vi "SR830 sweep update tw temporary 4.vi"() -> ()   [LabVIEW 2015]
uses:
  magnetometers/smi/labview/CPM20Software/SmartMotor.llb/SM Config.ctl
  magnetometers/smi/labview/CPM20Software/SmartMotor.llb/SM MotorConfig.ctl
  <vilib>/Analysis/1siggen.llb/Ramp Pattern by Samples.vi
  <vilib>/Utility/file.llb/Write To Spreadsheet File (DBL).vi
  Global vab.vi
  <vilib>/Analysis/NI_AALBase.lvlib
panel:
  in  "Laser lock":bool
  out "read buffer":string
  in  "USB relay com port":refnum<visa-resource-name>="COM5"
  in  "Back position (mm)":dbl=120.0
  in  "Back velocity (mm/sec)":dbl=1.0
  out "SM motor moving":bool
  out "Lock data":dbl[][](array[numeric])=[[0.0, -9.2798e-08], [0.0, -9.27907e-08], [0.0, -9.27762e-08], [0.00508, -9.27762e-08], [0.03048, -9.27762e-08], [0.10668000000000001, -9.27762e-08], [0.17272, -9.27762e-08], [0.23368, -9.27762e-08], [0.28956000000000004, -9.27253e-08], [0.34036000000000005, -9.27253e-08], [0.39116, -9.27325e-08], [0.43688, -9.27398e-08], [0.48768, -9.27398e-08], [0.5334, -9.27253e-08], [0.5842, -9.2718e-08], [0.635, -9.27253e-08], [0.6807200000000001, -9.27253e-08], [0.73152, -9.27107e-08], [0.78232, -9.27034e-08], [0.8331200000000001, -9.2718e-08], [0.8839199999999999, -9.2718e-08], [0.93472, -9.27398e-08], [0.9855200000000001, -9.27253e-08], [1.0312400000000002, -9.2718e-08], [1.08204, -9.27253e-08], [1.12776, -9.27253e-08], [1.17856, -9.2718e-08], [1.22936, -9.2718e-08], [1.27508, -9.2718e-08], [1.3258800000000002, -9.27253e-08], [1.3766800000000001, -9.27471e-08], [1.4224, -9.27544e-08], [1.4731999999999998, -9.27471e-08], [1.524, -9.27398e-08], [1.56972, -9.27398e-08], [1.6256000000000002, -9.27471e-08], [1.6713200000000001, -9.27398e-08], [1.72212, -9.27398e-08], [1.7729199999999998, -9.27398e-08], [1.81864, -9.27398e-08], [1.86944, -9.27325e-08], [1.91516, -9.27398e-08], [1.9659600000000002, -9.27471e-08], [2.01168, -9.27325e-08], [2.0624800000000003, -9.27325e-08], [2.11836, -9.27544e-08], [2.16408, -9.27398e-08], [2.21488, -9.27398e-08], [2.2606, -9.27253e-08], [2.3114, -9.27253e-08], [2.35712, -9.2718e-08], [2.40792, -9.27253e-08], [2.45364, -9.27253e-08], [2.50444, -9.2718e-08], [2.55524, -9.27398e-08], [2.60604, -9.27325e-08], [2.6568400000000003, -9.26962e-08], [2.70764, -9.26743e-08], [2.7584400000000002, -9.26889e-08], [2.8092400000000004, -9.2718e-08], [2.8600399999999997, -9.2718e-08], [2.90576, -9.2718e-08], [2.9514799999999997, -9.2718e-08], [3.00228, -9.2718e-08], [3.048, -9.26889e-08], [3.0987999999999998, -9.26816e-08], [3.1496, -9.27034e-08], [3.2004, -9.2718e-08], [3.24612, -9.2718e-08], [3.29184, -9.2718e-08], [3.3426400000000003, -9.2718e-08], [3.3934400000000005, -9.27107e-08], [3.44424, -9.26889e-08], [3.49504, -9.26598e-08], [3.5509199999999996, -9.26743e-08], [3.59664, -9.27107e-08], [3.64744, -9.2718e-08], [3.6982399999999997, -9.27107e-08], [3.73888, -9.2718e-08], [3.79476, -9.27107e-08], [3.84048, -9.27325e-08], [3.89128, -9.27253e-08], [3.9370000000000003, -9.27253e-08], [3.9878, -9.2718e-08], [4.03352, -9.27107e-08], [4.08432, -9.2718e-08], [4.13512, -9.2718e-08], [4.18084, -9.27107e-08], [4.23164, -9.27107e-08], [4.28244, -9.2718e-08], [4.33832, -9.27398e-08], [4.37896, -9.27398e-08], [4.42976, -9.27253e-08], [4.48056, -9.2718e-08], [4.52628, -9.2718e-08], [4.5770800000000005, -9.2718e-08], [4.6228, -9.27034e-08], [4.6736, -9.26962e-08], [4.7244, -9.26889e-08], [4.7701199999999995, -9.26962e-08], [4.82092, -9.27034e-08], [4.87172, -9.2718e-08], [4.91744, -9.2718e-08], [4.97332, -9.27107e-08], [5.0038, -9.27107e-08], [0.0, -9.27253e-08], [4.99872, -9.27253e-08], [4.99872, -9.27253e-08], [4.99872, -9.2718e-08], [4.94284, -9.27034e-08], [4.86156, -9.26889e-08], [4.8006, -9.26743e-08], [4.74472, -9.26743e-08], [4.69392, -9.26962e-08], [4.643120000000001, -9.27034e-08], [4.59232, -9.26962e-08], [4.5466, -9.27034e-08], [4.4958, -9.27107e-08], [4.45008, -9.27034e-08], [4.40436, -9.26962e-08], [4.35356, -9.26816e-08], [4.30784, -9.27034e-08], [4.2621199999999995, -9.26962e-08], [4.2164, -9.26889e-08], [4.17068, -9.27034e-08], [4.11988, -9.27034e-08], [4.07924, -9.27034e-08], [4.02336, -9.26962e-08], [3.97764, -9.26598e-08], [3.9268400000000003, -9.26816e-08], [3.88112, -9.27034e-08], [3.8354, -9.26889e-08], [3.78968, -9.26962e-08], [3.73888, -9.26889e-08], [3.6931599999999998, -9.26889e-08], [3.64744, -9.27107e-08], [3.59664, -9.2718e-08], [3.5559999999999996, -9.27471e-08], [3.5052, -9.27471e-08], [3.45948, -9.27398e-08], [3.4137600000000003, -9.2718e-08], [3.36804, -9.2718e-08], [3.3223200000000004, -9.27253e-08], [3.27152, -9.27325e-08], [3.2258, -9.27253e-08], [3.1800800000000002, -9.27253e-08], [3.13436, -9.2718e-08], [3.0734, -9.27107e-08], [3.03276, -9.26816e-08], [2.98704, -9.26962e-08], [2.9362399999999997, -9.27034e-08], [2.89052, -9.2718e-08], [2.84988, -9.2718e-08], [2.7940000000000005, -9.26671e-08], [2.7533600000000003, -9.26743e-08], [2.70764, -9.26962e-08], [2.6568400000000003, -9.27107e-08], [2.61112, -9.27034e-08], [2.5654, -9.27034e-08], [2.5146, -9.26816e-08], [2.46888, -9.26743e-08], [2.4231599999999998, -9.26816e-08], [2.37744, -9.27034e-08], [2.3266400000000003, -9.27107e-08], [2.28092, -9.27034e-08], [2.2352, -9.2718e-08], [2.1844, -9.2718e-08], [2.13868, -9.27034e-08], [2.0929599999999997, -9.27034e-08], [2.04216, -9.27034e-08], [1.99136, -9.27034e-08], [1.95072, -9.26962e-08], [1.905, -9.26816e-08], [1.85928, -9.26816e-08], [1.8084799999999999, -9.26889e-08], [1.7627599999999999, -9.26889e-08], [1.7170400000000001, -9.26962e-08], [1.6662400000000002, -9.27034e-08], [1.62052, -9.27107e-08], [1.5748, -9.2718e-08], [1.52908, -9.2718e-08], [1.4731999999999998, -9.2718e-08], [1.4325599999999998, -9.27107e-08], [1.38684, -9.2718e-08], [1.3360400000000001, -9.27107e-08], [1.28524, -9.26962e-08], [1.2446, -9.26962e-08], [1.19888, -9.26962e-08], [1.14808, -9.26962e-08], [1.10236, -9.27107e-08], [1.05664, -9.27107e-08], [1.01092, -9.27253e-08], [0.96012, -9.27253e-08], [0.9144, -9.2718e-08], [0.8636, -9.2718e-08], [0.81788, -9.27253e-08], [0.77216, -9.2718e-08], [0.72644, -9.2718e-08], [0.67564, -9.27034e-08], [0.62992, -9.27107e-08], [0.5791200000000001, -9.27253e-08], [0.52832, -9.2718e-08], [0.48768, -9.2718e-08], [0.44195999999999996, -9.27034e-08], [0.39624, -9.26962e-08], [0.35052000000000005, -9.27034e-08], [0.30988, -9.26889e-08], [0.26416, -9.26743e-08], [0.21844, -9.26889e-08], [0.17272, -9.26889e-08], [0.127, -9.26889e-08], [0.09652, -9.26889e-08], [0.04064, -9.26962e-08], [-0.00508, -9.26962e-08], [0.0, -9.27544e-08]]
  out "Last lock file":path=path "C:/Shoujun/07272005/lock.008"
  in  "Save lock":bool
  out "Last sweep file":path=path "C:/Shoujun/06122015/scan002"
  in  "Save sweep":bool
  out "Ccurrent times":dbl
  in  "Moving times":dbl=1.0
  in  "Waiting time (s)":dbl=3.0
  in  "Stop motor":bool
  out "Motor position (mm)":dbl
  in  "SM setting":T1={"Acceleration (mm/sec^2)"=1000.0, "Velocity (mm/sec)"=2.0, "Position (mm)"=0.0} {"Position (mm)" format="%.3f"; "Velocity (mm/sec)" format="%.3f"; "Acceleration (mm/sec^2)" format="%.3f"}
  in  "SM Config":T2={"VISA Serial ref"="COM3", "Motor Config"={"DriveRatio (mm/rev)"=10.16, "PosLimit + (mm)"=200.0, "PosLimit - (mm)"=0.0, "EncoderRatio (count/rev)"=2000.0, "MotorType"=enum."SM17"}} {"Motor Config"."EncoderRatio (count/rev)" format="%.2f"; "Motor Config"."PosLimit - (mm)" format="%.3f"; "Motor Config"."PosLimit + (mm)" format="%.3f"; "Motor Config"."DriveRatio (mm/rev)" format="%.2f"}
  in  "Motor moving mode":u16(ring) items=["One-way", "Two-way"]
  out "Step time (ms)":u32
  out "Center Freq. (Hz)":dbl=1279.6242713207916 format="%#_8f"
  in  "DS345 parameters":T4={"Osc. Amp. (V)"=0.06, "Osc. Freq. (Hz)"=1140.0} {"Osc. Freq. (Hz)" min=0.001 max=250000.0 step=0.001 format="%.3f"; "Osc. Amp. (V)" min=0.0 max=0.1 step=0.001 format="%.3f"}
  out "Lock Chart":dbl(graph)
  in  "Lock":bool
  in  "Update":bool
  in  "Auto-phase":bool
  in  "Update Aux Outs":bool
  in  "Lock-in  \naux outs (V)":dbl[](array[numeric])=[3.0, 0.0, -3.0, 4.0]
  in  "stop":bool
  in  "Lock in parameters":T5={"Phase (deg)"=190.0, "TC"=7, "TC Multiplier"=5.0} {"TC Multiplier" min=0.0 max=10.0 step=1.0 format="%.2f"; "TC" items=["10 µs", "30 µs", "100 µs", "300 µs", "1 ms", "3 ms", "10 ms", "30 ms", "100 ms", "300 ms", "1 s", "3 s", "10 s", "30 s", "100 s", "300 s", "1 ks", "3 ks", "10 ks", "30 ks"]; "Phase (deg)" format="%.3f"}
  out "Sweep Fit Chart":dbl[][](graph)
  out "Best Fit Coefficients":dbl[][](array[numeric])=[[116.36223046164876, 1127.5591284236862, 2.415453805851806, 2.8898288492774762e-08, 1.3970935970960048e-10, -9.348733573586501e-08], [116.33952287251303, 1126.8840669250824, 92.71773761789645, 2.8818113222476787e-08, 1.0278120537649892e-10, 1.3998320692235225e-07]] format="%#_6p"
  out "Sweep fit data":dbl[][](array[numeric])=[[-9.278428993694947e-08, 1.2151206747589936e-07], [-9.257777429927783e-08, 1.2146574495873341e-07], [-9.237209921929236e-08, 1.2141607252254236e-07], [-9.216734571334164e-08, 1.2136297955084925e-07], [-9.196359932316975e-08, 1.2130639502797934e-07], [-9.176095032811043e-08, 1.2124624766638154e-07], [-9.155949396397681e-08, 1.2118246604883246e-07], [-9.13593306484252e-08, 1.211149787867336e-07], [-9.116056621249537e-08, 1.2104371469578182e-07], [-9.096331213794347e-08, 1.2096860299036584e-07], [-9.076768579988502e-08, 1.208895734981137e-07], [-9.057381071415596e-08, 1.2080655689608598e-07], [-9.038181678867532e-08, 1.2071948497018084e-07], [-9.019184057795565e-08, 1.2062829089938097e-07], [-9.000402553975253e-08, 1.2053290956653703e-07], [-8.98185222926743e-08, 1.20433277897436e-07], [-8.963548887338411e-08, 1.203293352299526e-07], [-8.945509099181811e-08, 1.2022102371511948e-07], [-8.92775022826158e-08, 1.2010828875197835e-07], [-8.910290455070839e-08, 1.1999107945808357e-07], [-8.893148800873977e-08, 1.1986934917752383e-07], [-8.876345150369997e-08, 1.1974305602829554e-07], [-8.859900272983336e-08, 1.1961216349080777e-07], [-8.843835842454211e-08, 1.1947664103921127e-07], [-8.828174454364171e-08, 1.193364648171232e-07], [-8.812939641193772e-08, 1.1919161835915823e-07], [-8.798155884468516e-08, 1.1904209335946764e-07], [-8.783848623506419e-08, 1.1888789048822932e-07], [-8.770044260236139e-08, 1.1872902025671231e-07], [-8.756770159508958e-08, 1.1856550393115542e-07], [-8.744054644281251e-08, 1.1839737449524304e-07], [-8.731926984997504e-08, 1.1822467766042538e-07], [-8.720417382457544e-08, 1.1804747292270706e-07], [-8.709556943406905e-08, 1.1786583466381296e-07], [-8.699377648046863e-08, 1.1767985329382321e-07], [-8.689912308622005e-08, 1.1748963643144947e-07], [-8.681194518209715e-08, 1.1729531011709283e-07], [-8.673258588809238e-08, 1.1709702005268066e-07], [-8.66613947780996e-08, 1.1689493286102198e-07], [-8.659872701911271e-08, 1.166892373560515e-07], [-8.654494237572095e-08, 1.1648014581385351e-07], [-8.650040407089468e-08, 1.162678952327797e-07], [-8.646547749444962e-08, 1.1605274856930732e-07], [-8.644052875118079e-08, 1.1583499593454794e-07], [-8.64259230414993e-08, 1.1561495573452977e-07], [-8.642202286851262e-08, 1.1539297573557164e-07], [-8.642918606689061e-08, 1.1516943403427588e-07], [-8.644776365058209e-08, 1.1494473990993435e-07], [-8.64780974785094e-08, 1.1471933453551767e-07], [-8.652051773979436e-08, 1.1449369152195575e-07], [-8.657534026286338e-08, 1.1426831726918777e-07], [-8.664286365595156e-08, 1.140437510965259e-07], [-8.672336629006395e-08, 1.138205651243217e-07], [-8.681710313934008e-08, 1.1359936387882222e-07], [-8.692430249797145e-08, 1.1338078359254025e-07], [-8.704516259729139e-08, 1.131654911735182e-07], [-8.717984815132624e-08, 1.129541828186175e-07], [-8.73284868638809e-08, 1.1274758224848306e-07], [-8.749116593502439e-08, 1.125464385451754e-07], [-8.766792860952055e-08, 1.123515235776711e-07], [-8.785877081417203e-08, 1.1216362900552807e-07], [-8.80636379350548e-08, 1.1198356285698996e-07], [-8.828242178904716e-08, 1.1181214568462754e-07], [-8.851495784672179e-08, 1.1165020630921665e-07], [-8.87610227653934e-08, 1.1149857717082398e-07], [-8.902033229172319e-08, 1.1135808931486821e-07], [-8.92925395926122e-08, 1.112295670500614e-07], [-8.957723407103051e-08, 1.1111382232439058e-07], [-8.987394071981971e-08, 1.1101164887441855e-07], [-9.018212006130215e-08, 1.1092381621188385e-07], [-9.050116871371693e-08, 1.108510635195627e-07], [-9.08304206171131e-08, 1.1079409353531224e-07], [-9.116914894146363e-08, 1.1075356650884374e-07], [-9.151656868858414e-08, 1.1073009431979129e-07], [-9.187183998717035e-08, 1.107242348477972e-07], [-9.22340720671979e-08, 1.1073648668542749e-07], [-9.260232788639432e-08, 1.107672842826178e-07], [-9.297562936787966e-08, 1.1081699360696361e-07], [-9.335296319478886e-08, 1.1088590839752084e-07], [-9.373328709516066e-08, 1.109742470809708e-07], [-9.411553653902002e-08, 1.1108215040820914e-07], [-9.449863175978703e-08, 1.1120967985690896e-07], [-9.488148500426463e-08, 1.1135681683171895e-07], [-9.526300790977496e-08, 1.1152346267888724e-07], [-9.564211890374562e-08, 1.117094395166938e-07], [-9.601775052031209e-08, 1.1191449186759197e-07], [-9.638885653034085e-08, 1.1213828906287883e-07], [-9.675441878561362e-08, 1.1238042837648129e-07], [-9.711345368460556e-08, 1.1264043883148628e-07], [-9.746501817608558e-08, 1.1291778561171267e-07], [-9.780821522736294e-08, 1.1321187500122058e-07], [-9.814219869602744e-08, 1.1352205976739033e-07], [-9.84661775570772e-08, 1.1384764489820865e-07], [-9.877941945096975e-08, 1.1418789360171566e-07], [-9.908125353194587e-08, 1.1454203347514908e-07], [-9.937107260954993e-08, 1.1490926275305287e-07], [-9.964833458923416e-08, 1.1528875654731036e-07], [-9.991256322995798e-08, 1.1567967299747591e-07], [-1.0016334824750823e-07, 1.1608115925663376e-07], [-1.0040034480166377e-07, 1.164923572460048e-07], [-1.0062327241316715e-07, 1.1691240912033472e-07], [-1.0083191336266948e-07, 1.173404623954193e-07], [-1.0102611062836781e-07, 1.177756746986579e-07], [-1.0120576542199472e-07, 1.1821721811300182e-07], [-1.0137083438423545e-07, 1.1866428309384035e-07], [-1.0152132650066499e-07, 1.191160819470443e-07], [-1.0165729979806487e-07, 1.1957185186439482e-07], [-1.0177885787867792e-07, 1.2003085751985298e-07], [-1.0188614634676502e-07, 1.2049239323648097e-07], [-1.0197934917793213e-07, 1.2095578473926653e-07], [-1.0205868507727816e-07, 1.2142039051361878e-07], [-1.0212440386764666e-07, 1.2188560279290256e-07], [-1.0217678294430411e-07, 1.223508482011107e-07], [-1.0221612382735416e-07, 1.228155880786833e-07], [-1.0224274883825146e-07, 1.232793185206537e-07], [-1.0225699792200032e-07, 1.2374157015680308e-07], [-1.0225922563209356e-07, 1.2420190770342955e-07], [-1.0224979829102574e-07, 1.2465992931576863e-07], [-1.0222909133534692e-07, 1.251152657691261e-07], [-1.0219748685073481e-07, 1.2556757949547977e-07], [-1.0215537129946893e-07, 1.2601656350075602e-07], [-1.0210313343999116e-07, 1.2646194018625233e-07], [-1.0204116243592457e-07, 1.269034600958256e-07], [-1.0196984614998213e-07, 1.2734090060854922e-07], [-1.0188956961660426e-07, 1.2777406459460899e-07], [-1.0180071368589654e-07, 1.2820277905029003e-07], [-1.0170365383046482e-07, 1.2862689372604844e-07], [-1.0159875910603566e-07, 1.2904627975987226e-07], [-1.014863912562747e-07, 1.2946082832644712e-07], [-1.0136690395194417e-07, 1.2987044931105887e-07], [-1.012406421544441e-07, 1.3027507001570074e-07], [-1.0110794159383338e-07, 1.3067463390350941e-07], [-1.0096912835159999e-07, 1.3106909938643534e-07], [-1.0082451853872258e-07, 1.3145843865995573e-07], [-1.0067441805991713e-07, 1.3184263658765976e-07], [-1.0051912245537246e-07, 1.3222168963767397e-07], [-1.0035891681173344e-07, 1.325956048721376e-07], [-1.0019407573457405e-07, 1.3296439899028532e-07], [-1.0002486337510369e-07, 1.3332809742513234e-07], [-9.985153350435836e-08, 1.3368673349328222e-07], [-9.967432962863503e-08, 1.3404034759698076e-07], [-9.949348514042729e-08, 1.343889864772119e-07], [-9.930922349960456e-08, 1.347327025163688e-07], [-9.912175844004607e-08, 1.350715530888238e-07], [-9.893129419738688e-08, 1.3540559995756362e-07], [-9.873802575395663e-08, 1.3573490871493906e-07], [-9.854213909739125e-08, 1.360595482655007e-07], [-9.834381148977033e-08, 1.3637959034884478e-07], [-9.814321174448147e-08, 1.3669510910037385e-07], [-9.794050050833378e-08, 1.3700618064788107e-07]] format="%#_6p"
  out "Sweep data":dbl[][](array[numeric])=[[1040.0, -9.17285e-08, 1.21029e-07], [1041.0738255033557, -9.19904e-08, 1.21277e-07], [1042.1476510067114, -9.20122e-08, 1.21306e-07], [1043.221476510067, -9.20268e-08, 1.2132e-07], [1044.2953020134228, -9.19831e-08, 1.21277e-07], [1045.3691275167785, -9.19758e-08, 1.21262e-07], [1046.4429530201342, -9.18303e-08, 1.21269e-07], [1047.5167785234898, -9.16557e-08, 1.21233e-07], [1048.5906040268455, -9.14592e-08, 1.21197e-07], [1049.6644295302012, -9.12628e-08, 1.21131e-07], [1050.7382550335572, -9.10227e-08, 1.21022e-07], [1051.8120805369128, -9.08117e-08, 1.20935e-07], [1052.8859060402685, -9.06152e-08, 1.20825e-07], [1053.9597315436242, -9.03897e-08, 1.20716e-07], [1055.03355704698, -9.0135e-08, 1.20578e-07], [1056.1073825503356, -8.9924e-08, 1.20462e-07], [1057.1812080536913, -8.97567e-08, 1.20389e-07], [1058.255033557047, -8.96111e-08, 1.20323e-07], [1059.3288590604027, -8.94511e-08, 1.20243e-07], [1060.4026845637584, -8.92619e-08, 1.20112e-07], [1061.476510067114, -8.90436e-08, 1.19931e-07], [1062.5503355704698, -8.88181e-08, 1.19763e-07], [1063.6241610738255, -8.86071e-08, 1.19603e-07], [1064.6979865771812, -8.84324e-08, 1.19443e-07], [1065.7718120805368, -8.82869e-08, 1.19327e-07], [1066.8456375838925, -8.81341e-08, 1.19144e-07], [1067.9194630872482, -8.78867e-08, 1.18941e-07], [1068.993288590604, -8.77194e-08, 1.1873e-07], [1070.0671140939598, -8.75593e-08, 1.18562e-07], [1071.1409395973155, -8.74502e-08, 1.18424e-07], [1072.2147651006712, -8.73192e-08, 1.18264e-07], [1073.288590604027, -8.72246e-08, 1.18097e-07], [1074.3624161073826, -8.71446e-08, 1.17995e-07], [1075.4362416107383, -8.70791e-08, 1.179e-07], [1076.510067114094, -8.69991e-08, 1.17769e-07], [1077.5838926174497, -8.69045e-08, 1.17602e-07], [1078.6577181208054, -8.68026e-08, 1.17369e-07], [1079.731543624161, -8.66571e-08, 1.17063e-07], [1080.8053691275168, -8.65844e-08, 1.16838e-07], [1081.8791946308725, -8.65043e-08, 1.16656e-07], [1082.9530201342282, -8.64825e-08, 1.16445e-07], [1084.0268456375838, -8.64388e-08, 1.16256e-07], [1085.1006711409395, -8.6417e-08, 1.16045e-07], [1086.1744966442952, -8.63806e-08, 1.15834e-07], [1087.248322147651, -8.63588e-08, 1.15594e-07], [1088.3221476510066, -8.63442e-08, 1.1539e-07], [1089.3959731543623, -8.63588e-08, 1.1515e-07], [1090.4697986577182, -8.64097e-08, 1.1499e-07], [1091.543624161074, -8.65043e-08, 1.14851e-07], [1092.6174496644296, -8.65407e-08, 1.14633e-07], [1093.6912751677853, -8.65844e-08, 1.14364e-07], [1094.765100671141, -8.66207e-08, 1.14109e-07], [1095.8389261744967, -8.66717e-08, 1.1384e-07], [1096.9127516778524, -8.67735e-08, 1.13571e-07], [1097.986577181208, -8.69118e-08, 1.13382e-07], [1099.0604026845638, -8.70646e-08, 1.13171e-07], [1100.1342281879195, -8.7181e-08, 1.12923e-07], [1101.2080536912752, -8.73265e-08, 1.12734e-07], [1102.2818791946308, -8.75084e-08, 1.1256e-07], [1103.3557046979865, -8.7683e-08, 1.12341e-07], [1104.4295302013422, -8.78285e-08, 1.12072e-07], [1105.503355704698, -8.80323e-08, 1.11883e-07], [1106.5771812080536, -8.82796e-08, 1.1173e-07], [1107.6510067114093, -8.85343e-08, 1.11592e-07], [1108.724832214765, -8.8738e-08, 1.1141e-07], [1109.7986577181207, -8.89927e-08, 1.11199e-07], [1110.8724832214766, -8.92546e-08, 1.11075e-07], [1111.9463087248323, -8.9582e-08, 1.1101e-07], [1113.020134228188, -8.99386e-08, 1.11002e-07], [1114.0939597315437, -9.02514e-08, 1.10981e-07], [1115.1677852348994, -9.05789e-08, 1.10901e-07], [1116.241610738255, -9.08917e-08, 1.10806e-07], [1117.3154362416108, -9.12191e-08, 1.10777e-07], [1118.3892617449665, -9.15975e-08, 1.10821e-07], [1119.4630872483222, -9.19904e-08, 1.1085e-07], [1120.5369127516778, -9.23615e-08, 1.10886e-07], [1121.6107382550335, -9.2718e-08, 1.10871e-07], [1122.6845637583892, -9.30454e-08, 1.10893e-07], [1123.758389261745, -9.3431e-08, 1.11002e-07], [1124.8322147651006, -9.3773e-08, 1.11046e-07], [1125.9060402684563, -9.41295e-08, 1.11082e-07], [1126.979865771812, -9.44933e-08, 1.11213e-07], [1128.0536912751677, -9.48717e-08, 1.11366e-07], [1129.1275167785234, -9.52136e-08, 1.11483e-07], [1130.2013422818793, -9.55774e-08, 1.11628e-07], [1131.275167785235, -9.59412e-08, 1.11883e-07], [1132.3489932885907, -9.63632e-08, 1.1213e-07], [1133.4228187919464, -9.67343e-08, 1.12399e-07], [1134.496644295302, -9.70836e-08, 1.12669e-07], [1135.5704697986578, -9.74401e-08, 1.12938e-07], [1136.6442953020135, -9.78184e-08, 1.13302e-07], [1137.7181208053692, -9.81458e-08, 1.13556e-07], [1138.7919463087248, -9.84296e-08, 1.13833e-07], [1139.8657718120805, -9.87279e-08, 1.14168e-07], [1140.9395973154362, -9.90044e-08, 1.14451e-07], [1142.013422818792, -9.92809e-08, 1.14844e-07], [1143.0872483221476, -9.96083e-08, 1.1523e-07], [1144.1610738255033, -9.98994e-08, 1.15695e-07], [1145.234899328859, -1.00161e-07, 1.16103e-07], [1146.3087248322147, -1.00423e-07, 1.16503e-07], [1147.3825503355704, -1.00649e-07, 1.16925e-07], [1148.456375838926, -1.00831e-07, 1.17398e-07], [1149.5302013422818, -1.00998e-07, 1.17762e-07], [1150.6040268456377, -1.01151e-07, 1.1814e-07], [1151.6778523489934, -1.01311e-07, 1.18555e-07], [1152.751677852349, -1.01464e-07, 1.19013e-07], [1153.8255033557048, -1.01616e-07, 1.19494e-07], [1154.8993288590605, -1.0174e-07, 1.20003e-07], [1155.9731543624162, -1.01893e-07, 1.20505e-07], [1157.0469798657718, -1.0198e-07, 1.20956e-07], [1158.1208053691275, -1.02053e-07, 1.21408e-07], [1159.1946308724832, -1.02119e-07, 1.21873e-07], [1160.268456375839, -1.02191e-07, 1.22353e-07], [1161.3422818791946, -1.02242e-07, 1.22834e-07], [1162.4161073825503, -1.02249e-07, 1.23248e-07], [1163.489932885906, -1.02213e-07, 1.23656e-07], [1164.5637583892617, -1.02184e-07, 1.241e-07], [1165.6375838926174, -1.02213e-07, 1.24587e-07], [1166.711409395973, -1.02242e-07, 1.25133e-07], [1167.7852348993288, -1.02213e-07, 1.25628e-07], [1168.8590604026845, -1.02199e-07, 1.2605e-07], [1169.9328859060402, -1.02155e-07, 1.26523e-07], [1171.006711409396, -1.02097e-07, 1.26966e-07], [1172.0805369127518, -1.02038e-07, 1.27425e-07], [1173.1543624161075, -1.01966e-07, 1.27847e-07], [1174.2281879194632, -1.01864e-07, 1.28269e-07], [1175.3020134228188, -1.01733e-07, 1.2864e-07], [1176.3758389261745, -1.01587e-07, 1.28953e-07], [1177.4496644295302, -1.01493e-07, 1.29382e-07], [1178.523489932886, -1.01391e-07, 1.29869e-07], [1179.5973154362416, -1.01296e-07, 1.30372e-07], [1180.6711409395973, -1.01209e-07, 1.30801e-07], [1181.744966442953, -1.01064e-07, 1.31223e-07], [1182.8187919463087, -1.00889e-07, 1.31616e-07], [1183.8926174496644, -1.00751e-07, 1.31965e-07], [1184.96644295302, -1.00583e-07, 1.32343e-07], [1186.0402684563758, -1.00423e-07, 1.327e-07], [1187.1140939597315, -1.00241e-07, 1.33049e-07], [1188.1879194630872, -1.00038e-07, 1.33318e-07], [1189.2617449664428, -9.98411e-08, 1.33631e-07], [1190.3355704697988, -9.96374e-08, 1.33929e-07], [1191.4093959731545, -9.94337e-08, 1.3425e-07], [1192.4832214765102, -9.92591e-08, 1.34592e-07], [1193.5570469798658, -9.90553e-08, 1.34963e-07], [1194.6308724832215, -9.88589e-08, 1.35268e-07], [1195.7046979865772, -9.86188e-08, 1.35545e-07], [1196.778523489933, -9.84296e-08, 1.35916e-07], [1197.8523489932886, -9.82768e-08, 1.36345e-07], [1198.9261744966443, -9.8124e-08, 1.36789e-07], [1200.0, -9.79639e-08, 1.37225e-07]]
  out "Sweep Chart":dbl[][](graph)
  in  "Sweep":bool
  in  "Sweep frequency":T6={"Start Freq. (Hz)"=1100.0, "Stop Freq. (Hz)"=1420.0, "# of Steps"=100} {"Stop Freq. (Hz)" min=0.0 max=3000.0 step=0.001 format="%.3f"; "Start Freq. (Hz)" min=0.0 max=3000.0 step=0.001 format="%.3f"}
  in  "SRS DS345 GPIB address":string="0:19"
  in  "Lock-in GPIB address":string="0:9"
  # "width              center freq.        phase            amplitude        linear bkgd         cont bkgd\n        (Hz)                    (Hz)                (deg.)                (A)                   (A)                     (A)"
  # "X"
  # "Y"
  # "SM motor setting"
  # "(Tic count, position, signal)"
  # "Remote USB for FM"
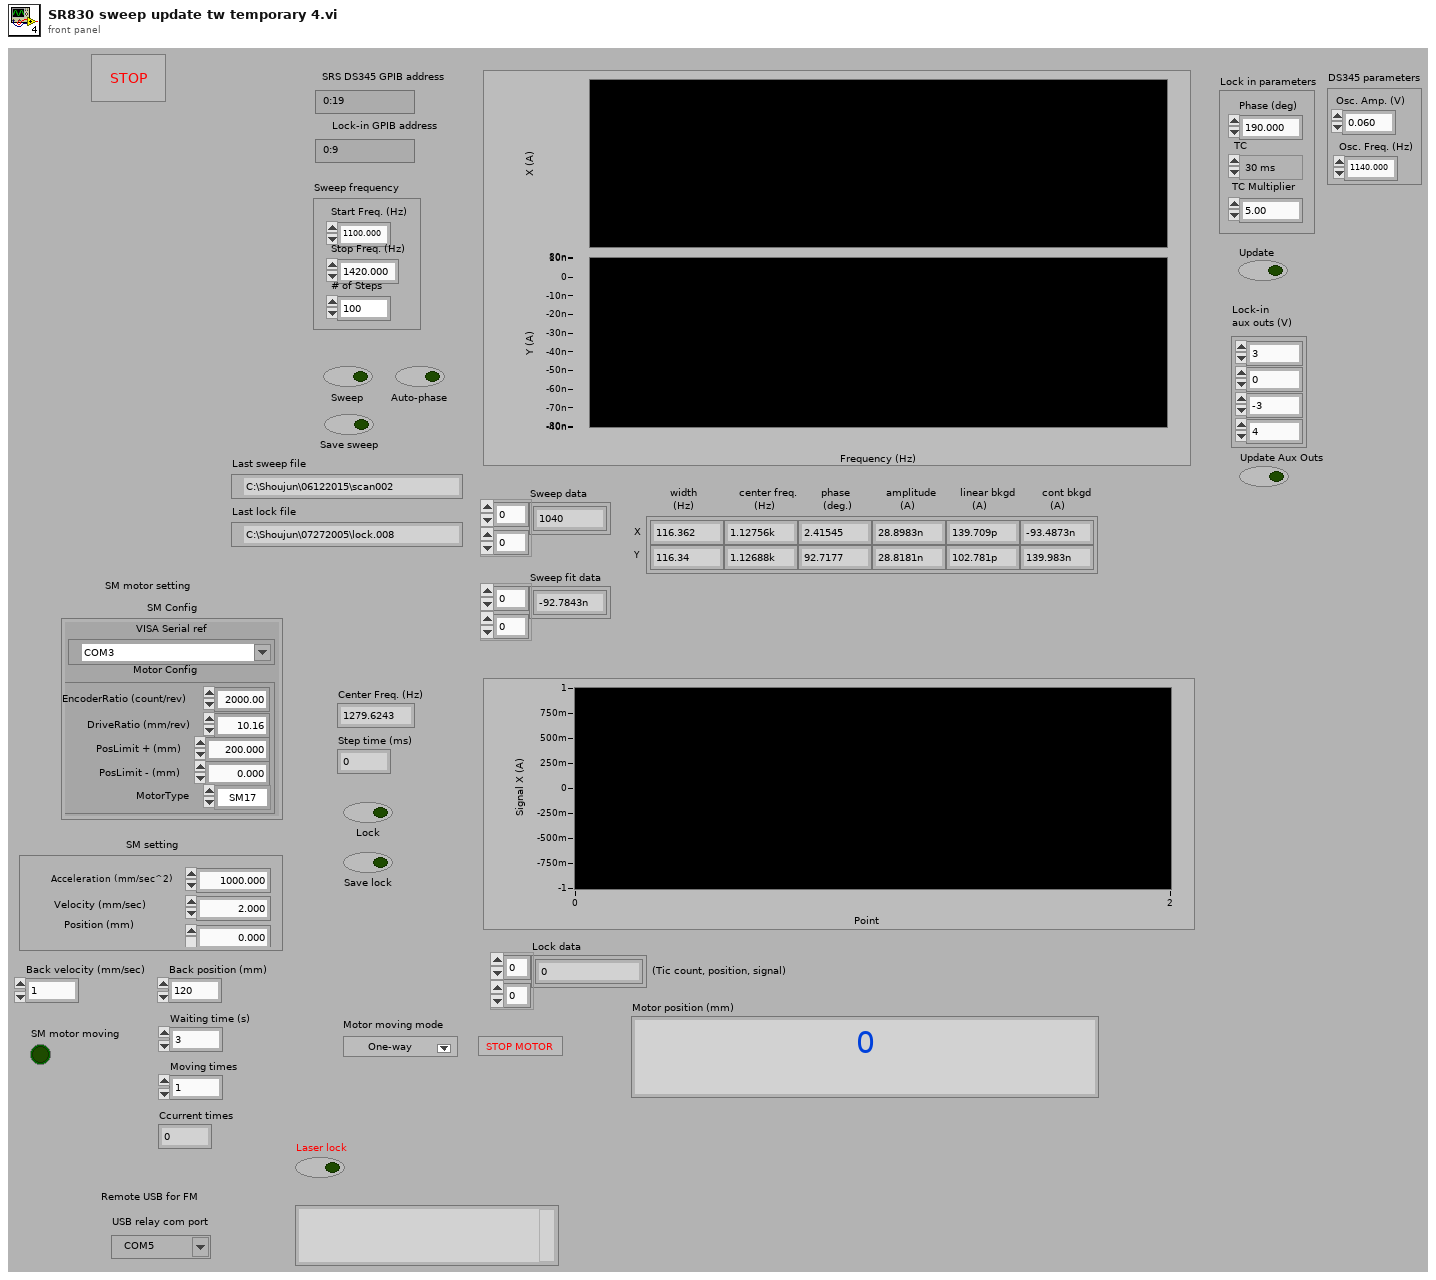
[diagram p1: front panel]
types:
  T1 = cluster{"Acceleration (mm/sec^2)":dbl, "Velocity (mm/sec)":dbl, "Position (mm)":dbl}
  T2 = typedef "SM Config.ctl" = cluster{"VISA Serial ref":refnum<visa-resource-name>, "Motor Config":T3}
  T3 = typedef "SM MotorConfig.ctl" = cluster{"DriveRatio (mm/rev)":dbl, "PosLimit + (mm)":dbl, "PosLimit - (mm)":dbl, "EncoderRatio (count/rev)":dbl, "MotorType":enum16{"SM17", "SM23", "SM34", "SM42", "SM56"}}
  T4 = cluster{"Osc. Amp. (V)":dbl, "Osc. Freq. (Hz)":dbl}
  T5 = cluster{"Phase (deg)":dbl, "TC":i32, "TC Multiplier":dbl}
  T6 = cluster{"Start Freq. (Hz)":dbl, "Stop Freq. (Hz)":dbl, "# of Steps":u16}
  T7 = typedef "SM Status.ctl" = cluster{"Trajectory In Progress":bool, "(+) Pos Limit":bool, "(-) Pos Limit":bool, "Index Report Available":bool, "Wraparound":bool, "Position Error":bool, "Excessive Temp":bool, "Motor off":bool}
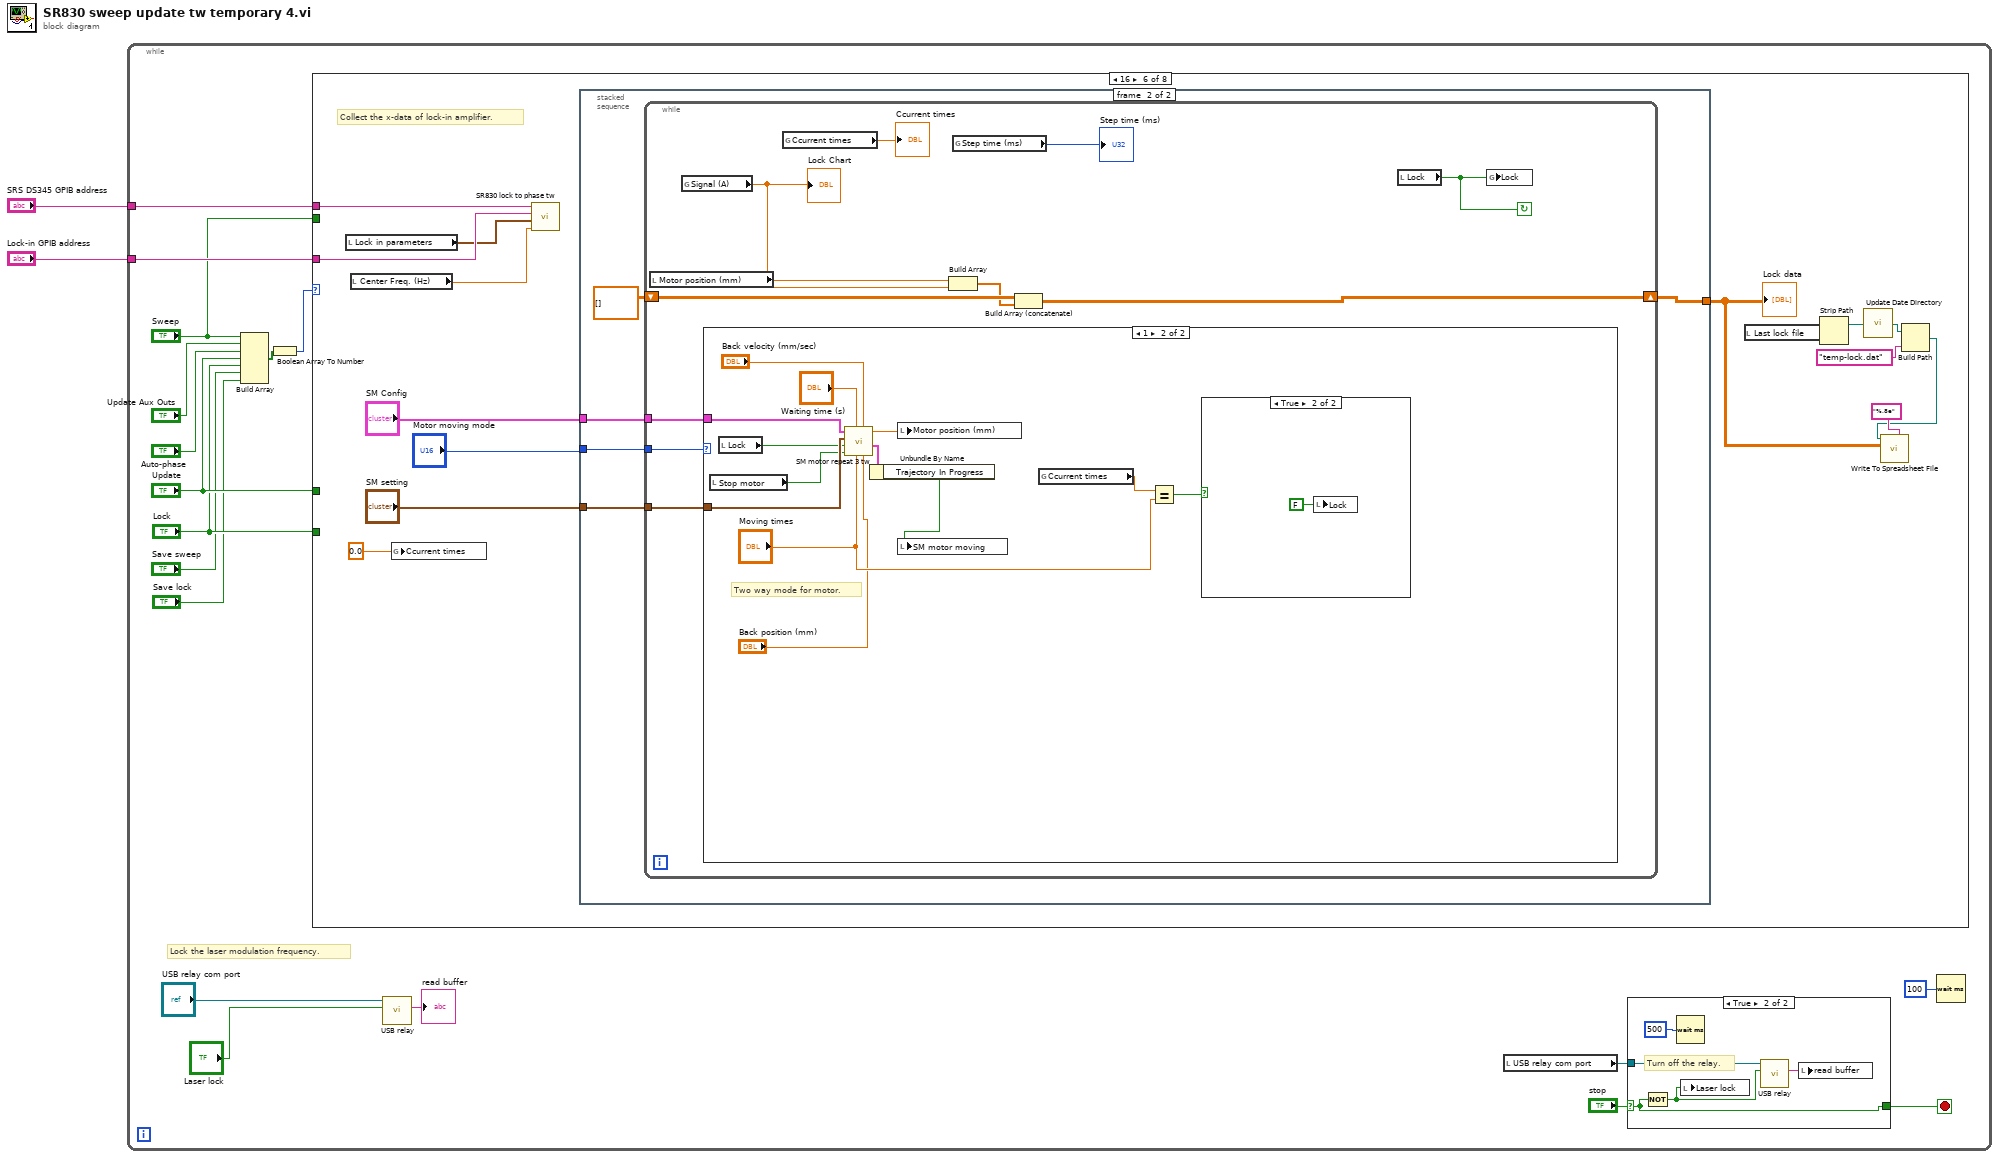
[diagram p0: block diagram]
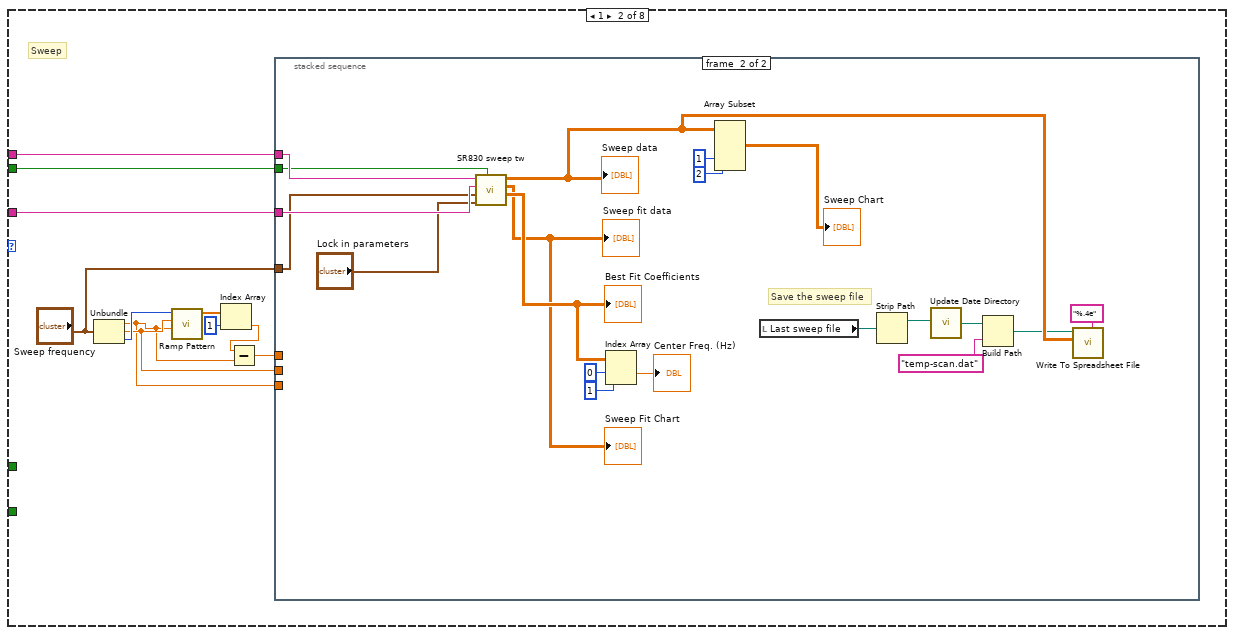
[diagram p4: hidden frame]
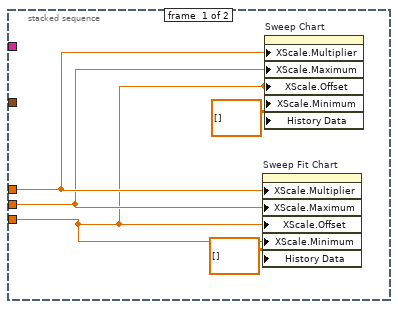
[diagram p5: hidden frame]
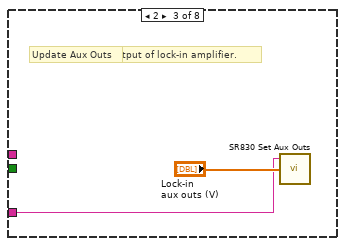
[diagram p6: hidden frame]
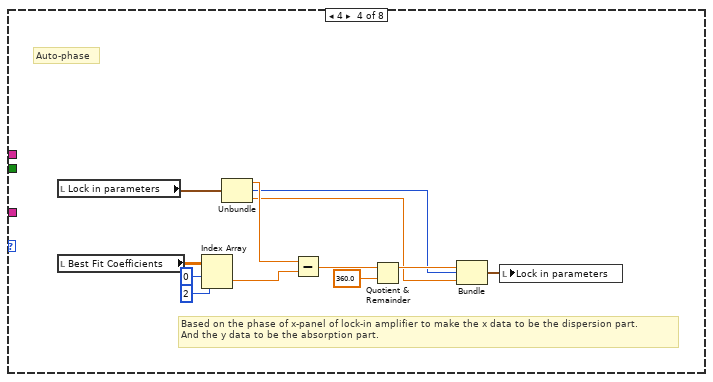
[diagram p7: hidden frame]
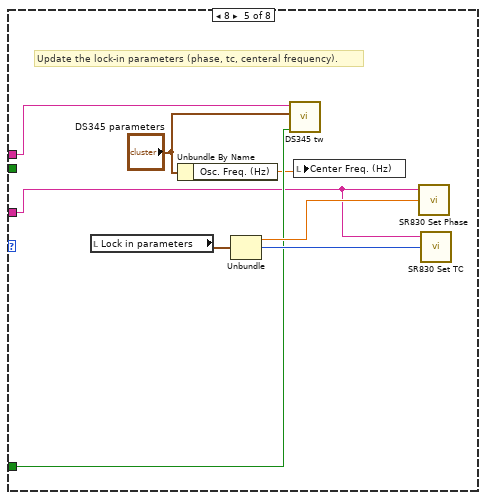
[diagram p8: hidden frame]
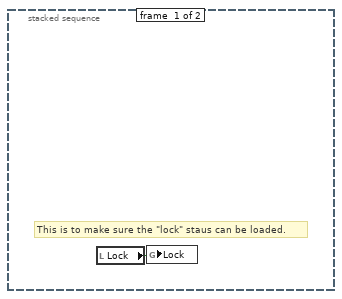
[diagram p9: hidden frame]
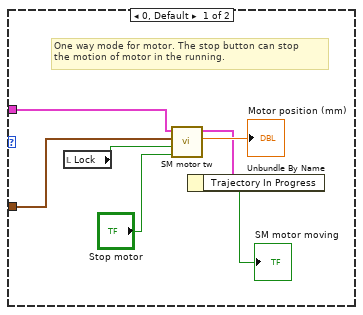
[diagram p10: hidden frame]
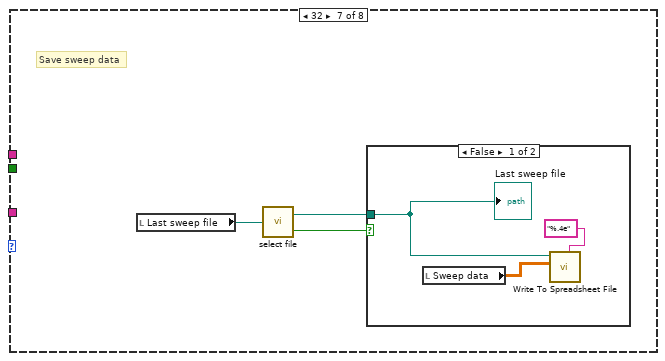
[diagram p12: hidden frame]
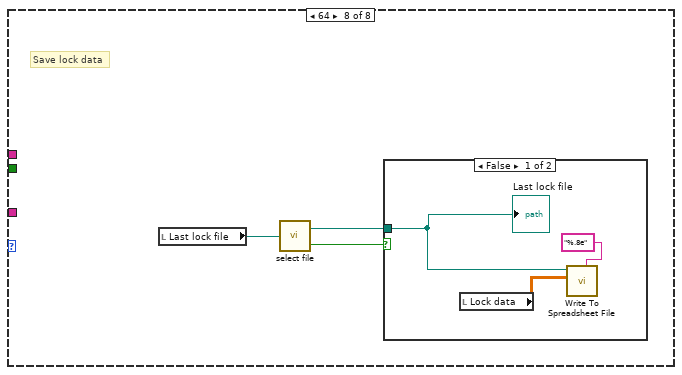
[diagram p14: hidden frame]
diagram:
  n1 = while {
    tunnel: "SRS DS345 GPIB address" -> [w19]
    tunnel: "Lock-in GPIB address" -> [w18]
    stop <- w4 stop-if-true
    # "Lock the laser modulation frequency."
    n2 = Build Array("Sweep", "Update Aux Outs", "Auto-phase", "Update", "Lock", "Save sweep", "Save lock") -> (w16:bool[])
    n3 = Boolean Array To Number(Boolean array=w16) -> (number=w15:u32)
    n4 = case shown="16" w15 {
      tunnel: w19 -> [_ w30 _ _ w81 w99 _ _]
      tunnel: w18 -> [_ w29 w63 _ w79 w98 _ _]
      tunnel: "Update" -> [_ _ _ _ w80 _ _ _]
      tunnel: "Lock" -> [_ _ _ _ _ _ _ _]
      tunnel: "Sweep" -> [_ w27 _ _ _ _ _ _]
      frame 0, Default {
      }
      frame 1 {
        # "Sweep"
        n5 = Unbundle("Sweep frequency") -> ("Start Freq. (Hz)"=w31:dbl, "Stop Freq. (Hz)"=w32:dbl, "# of Steps"=w37:u16)
        n6 = call-poly <vilib>:"Ramp Pattern.vi"("start"=w31, "end"=w32, "samples"=w37) -> ("Ramp Pattern"=w36:dbl[])  [unwired: 7 in, 1 out]
        n7 = Index Array(array=w36, index=1) -> (element=w34:dbl)
        n8 = Subtract(x=w34, y=w31) -> (x-y=w33:dbl)
        n9 = stacked-sequence {
          tunnel: w33 -> [w41 _]
          tunnel: w32 -> [w40 _]
          tunnel: w31 -> [w39 _]
          tunnel: w30 -> [_ w62]
          tunnel: w29 -> [_ w61]
          tunnel: "Sweep frequency" -> [_ w60]
          tunnel: w27 -> [_ w54]
          frame #0 {
            n10 = property on="Sweep Fit Chart" class="WFChart (strict)"("XScale.Multiplier"=w41, "XScale.Maximum"=w40, "XScale.Offset"=w39, "XScale.Minimum"=w39, "History Data"=dbl[][] []) -> ()  [unwired: 2 in, 2 out]
            n11 = property on="Sweep Chart" class="WFChart (strict)"("XScale.Multiplier"=w41, "XScale.Maximum"=w40, "XScale.Offset"=w39, "XScale.Minimum"=w39, "History Data"=dbl[][] []) -> ()  [unwired: 2 in, 2 out]
          }
          frame #1 {
            # "Save the sweep file"
            n12 = call "SR830 sweep tw.vi"("Sweep"=w54, "Lock in parameters"="Lock in parameters", "Sweep frequency"=w60, "Lock-in GPIB address"=w61, "SRS DS345 GPIB address"=w62) -> ("Best Fit Coefficients"=w56:dbl[][], "Sweep fit data"=→"Sweep fit data" →"Sweep Fit Chart":dbl[][], "Sweep data"=w45:dbl[][])  [unwired: 2 out]
            "Sweep data" <- w45
            "Best Fit Coefficients" <- w56
            n13 = Index Array(array=w56, index (row)=0, index (col)=1 ("disabled index (col)")) -> (element=→"Center Freq. (Hz)":dbl)
            n14 = Array Subset(array=w45, index (col)=1 ("index"), length (col)=2 ("length")) -> (→"Sweep Chart":dbl[][])  [unwired: 2 in]
            n15 = local read "Last sweep file"() -> (w44:path)
            n16 = Strip Path(path=w44) -> (stripped path=w47:path)  [unwired: 1 out]
            n17 = call "Update Date Directory.vi"("input path"=w47) -> ("output path"=w46:path)
            n18 = Build Path(base path=w46, name or relative path="temp-scan.dat") -> (appended path=w43:path)
            n19 = call-poly <vilib>:"Write To Spreadsheet File.vi"("format (%.3f)"="%.4e", "2D data"=w45, "file path (dialog if empty)"=w43) -> ()  [unwired: 3 in, 3 out]
          }
        }
      }
      frame 2 {
        # "Update Aux Outs"
        # "Change the aux output of lock-in amplifier."
        n20 = call "SR830 Set Aux Outs.vi"("Output Voltages (V)"="Lock-in  \naux outs (V)", "GPIB address"=w63) -> ()  [unwired: 1 in, 3 out]
      }
      frame 4 {
        # "Based on the phase of x-panel of lock-in amplifier to make the x data to be the dispersion part.\nAnd the y data to be the absorption part."
        # "Auto-phase"
        n21 = local read "Lock in parameters"() -> (w70:T5)
        n22 = local read "Best Fit Coefficients"() -> (w76:dbl[][])
        n23 = Index Array(array=w76, index (row)=0, index (col)=2 ("disabled index (col)")) -> (element=w73:dbl)
        n24 = Unbundle(w70) -> ("Phase (deg)"=w69:dbl, "TC"=w67:i32, "TC Multiplier"=w66:dbl)
        n25 = Subtract(x=w69, y=w73) -> (x-y=w72:dbl)
        n26 = Quotient & Remainder(x=w72, y=360.0) -> (x-y*floor(x/y)=w68:dbl)  [unwired: 1 out]
        n27 = Bundle(w68, "TC"=w67, "TC Multiplier"=w66) -> (w65:cluster{dbl, "TC":i32, "TC Multiplier":dbl})  [unwired: 1 out]
        n28 = local write "Lock in parameters"(w65) -> ()
      }
      frame 8 {
        # "Update the lock-in parameters (phase, tc, centeral frequency)."
        n29 = local read "Lock in parameters"() -> (w84:T5)
        n30 = Unbundle By Name("DS345 parameters") -> ("Osc. Freq. (Hz)"=w77:dbl)
        n31 = Unbundle(w84) -> ("Phase (deg)"=w83:dbl, "TC"=w82:i32)  [unwired: 1 out]
        n32 = call "DS345 tw.vi"("Update"=w80, "Cluster"="DS345 parameters", "SRS DS345 GPIB address"=w81) -> ()  [unwired: 9 out]
        n33 = local write "Center Freq. (Hz)"(w77) -> ()
        n34 = call "SR830 Set Phase.vi"("Phase (deg)"=w83, "GPIB address"=w79) -> ()  [unwired: 2 in, 2 out]
        n35 = call "SR830 Set TC.vi"("time constant\n(10 µs : 0)"=w82, "GPIB address"=w79) -> ()  [unwired: 1 in, 3 out]
      }
      frame 16 {
        # "Collect the x-data of lock-in amplifier."
        n36 = local read "Lock in parameters"() -> (w97:T5)
        n37 = local read "Center Freq. (Hz)"() -> (w92:dbl)
        n38 = global write "Global vab.vi" "Ccurrent times"(0.0 ("Ccurrent times")) -> ()
        n39 = call "SR830 lock to phase tw.vi"("Osc. Freq. (Hz)"=w92, "Lock in parameters"=w97, "Lock-in GPIB address"=w98, "SRS DS345 GPIB address"=w99) -> ()  [unwired: 1 in, 6 out]
        n40 = stacked-sequence {
          tunnel: "Motor moving mode" -> [_ w105]
          tunnel: "SM Config" -> [_ w104]
          tunnel: "SM setting" -> [_ w103]
          tunnel: [_ w101] -> w86
          frame #0 {
            # "This is to make sure the \"lock\" staus can be loaded."
            n41 = local read "Lock"() -> (w100:bool)
            n42 = global write "Global vab.vi" "Lock"(w100) -> ()
          }
          frame #1 {
            n43 = while {
              tunnel: w105 -> [w114]
              tunnel: w104 -> [w113]
              tunnel: w103 -> [w112]
              shift-right: [w107] -> w101
              shift-left: dbl[][] [] -> [w108]
              stop <- w115 continue-if-true
              n44 = local read "Motor position (mm)"() -> (w109:dbl)
              n45 = global read "Global vab.vi" "Signal (A)"() -> (w110:dbl)
              "Lock Chart" <- w110
              n46 = case shown="1" w114 {
                tunnel: w113 -> [w123 w136]
                tunnel: w112 -> [w122 w135]
                frame 0, Default {
                  # "One way mode for motor. The stop button can stop\nthe motion of motor in the running."
                  n47 = local read "Lock"() -> (w119:bool)
                  n48 = call "SM motor tw.vi"("SM Config"=w123, "SM setting"=w122, "Move"=w119, "Stop motion"="Stop motor") -> ("Status"=w118:T7, "Position (mm)"=→"Motor position (mm)":dbl)  [unwired: 5 out]
                  n49 = Unbundle By Name(w118) -> ("Trajectory In Progress"=→"SM motor moving":bool)
                }
                frame 1 {
                  # "Two way mode for motor."
                  n50 = local read "Stop motor"() -> (w131:bool)
                  n51 = local read "Lock"() -> (w132:bool)
                  n52 = call "SM motor repeat 3 tw.vi"("Back position (mm)"="Back position (mm)", "Back velocity (mm/sec)"="Back velocity (mm/sec)", "Moving times"="Moving times", "Waiting time (s)"="Waiting time (s)", "Stop motion"=w131, "Move"=w132, "SM setting"=w135, "SM Config"=w136) -> ("Status"=w130:T7, "Position (mm)"=w134:dbl)  [unwired: 2 in]
                  n53 = Unbundle By Name(w130) -> ("Trajectory In Progress"=w129:bool)
                  n54 = local write "Motor position (mm)"(w134) -> ()
                  n55 = local write "SM motor moving"(w129) -> ()
                  n56 = global read "Global vab.vi" "Ccurrent times"() -> (w128:dbl)
                  n57 = Equal?(x=w128, y="Moving times") -> (x = y?=w126:bool)
                  n58 = case shown="True" w126 {
                    frame False {
                    }
                    frame True {
                      n59 = local write "Lock"(FALSE ("Lock")) -> ()
                    }
                  }
                }
              }
              n60 = global read "Global vab.vi" "Ccurrent times"() -> (→"Ccurrent times":dbl)
              n61 = Build Array(w109, w110) -> (w106:dbl[])
              n62 = global read "Global vab.vi" "Step time (ms)"() -> (→"Step time (ms)":u32)
              n63 = Build Array (concatenate)(w108, w106) -> (w107:dbl[][])
              n64 = local read "Lock"() -> (w115:bool)
              n65 = global write "Global vab.vi" "Lock"(w115) -> ()
            }
          }
        }
        "Lock data" <- w86
        n66 = local read "Last lock file"() -> (w91:path)
        n67 = Strip Path(path=w91) -> (stripped path=w90:path)  [unwired: 1 out]
        n68 = call "Update Date Directory.vi"("input path"=w90) -> ("output path"=w89:path)
        n69 = Build Path(base path=w89, name or relative path="temp-lock.dat") -> (appended path=w85:path)
        n70 = call-poly <vilib>:"Write To Spreadsheet File.vi"("format (%.3f)"="%.8e", "2D data"=w86, "file path (dialog if empty)"=w85) -> ()  [unwired: 3 in, 3 out]
      }
      frame 32 {
        # "Save sweep data"
        n71 = local read "Last sweep file"() -> (w140:path)
        n72 = call "select file.vi"("old path"=w140) -> ("new path"=w138:path, "cancelled"=w139:bool)
        n73 = case shown="False" w139 {
          tunnel: w138 -> [w141 _]
          frame False {
            n74 = local read "Sweep data"() -> (w142:dbl[][])
            n75 = call-poly <vilib>:"Write To Spreadsheet File.vi"("format (%.3f)"="%.4e", "2D data"=w142, "file path (dialog if empty)"=w141) -> ()  [unwired: 3 in, 3 out]
            "Last sweep file" <- w141
          }
          frame True {
          }
        }
      }
      frame 64 {
        # "Save lock data"
        n76 = local read "Last lock file"() -> (w144:path)
        n77 = call "select file.vi"("old path"=w144) -> ("new path"=w145:path, "cancelled"=w146:bool)
        n78 = case shown="False" w146 {
          tunnel: w145 -> [w148 _]
          frame False {
            n79 = local read "Lock data"() -> (w147:dbl[][])
            n80 = call-poly <vilib>:"Write To Spreadsheet File.vi"("format (%.3f)"="%.8e", "2D data"=w147, "file path (dialog if empty)"=w148) -> ()  [unwired: 3 in, 3 out]
            "Last lock file" <- w148
          }
          frame True {
          }
        }
      }
    }
    n81 = call "USB relay.vi"("Relay on"="Laser lock", "USB relay com port"="USB relay com port") -> ("read buffer"=→"read buffer":string)  [unwired: 9 in]
    n82 = local read "USB relay com port"() -> (w3:refnum<visa-resource-name>)
    n83 = case shown="True" "stop" {
      selector: "stop" -> [w21 w26]
      tunnel: [w21 w26] -> w4
      tunnel: w3 -> [_ w24]
      frame False {
      }
      frame True {
        # "Turn off the relay."
        n84 = Not(x=w26) -> (.not. x?=w23:bool)
        n85 = Wait (ms)(milliseconds to wait=u32 500) -> ()  [unwired: 1 out]
        n86 = local write "Laser lock"(w23) -> ()
        n87 = call "USB relay.vi"("Relay on"=w23, "USB relay com port"=w24) -> ("read buffer"=w22:string)  [unwired: 9 in]
        n88 = local write "read buffer"(w22) -> ()
      }
    }
    n89 = Wait (ms)(milliseconds to wait=u32 100) -> ()  [unwired: 1 out]
  }
